vi "SearchGlyphs.vi"(4 "Glyphs tree":refnum<vi>, 6 "DNL_Glyphs []":refnum<vi>, 7 "Reset position? (F)":bool, 8 "error in (no error)":errorcluster, 10 "Keyword":string, 11 "Glyph in":refnum<class "Glyph.lvclass">) -> (0 "error out":errorcluster, 3 "Glyph out":refnum<class "Glyph.lvclass">)   [LabVIEW 2020, in "Glyph.lvclass"]
uses:
  Glyph.lvclass
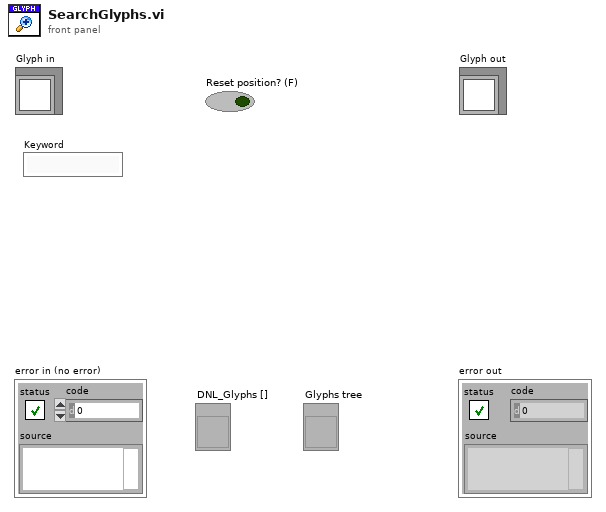
[diagram p1: front panel]
types:
  T1 = typedef "Graphic.ctl" = cluster{"Rectangle":cluster{"left":i16, "top":i16, "right":i16, "bottom":i16}, "Path":path, "Image":picture, "Filter":string, "FileName":string}
  T2 = typedef "Path&Icon.ctl" = cluster{"Rectangle":cluster{"left":i16, "top":i16, "right":i16, "bottom":i16}, "Path":path, "Image":picture, "Filter":string, "FileName":string}
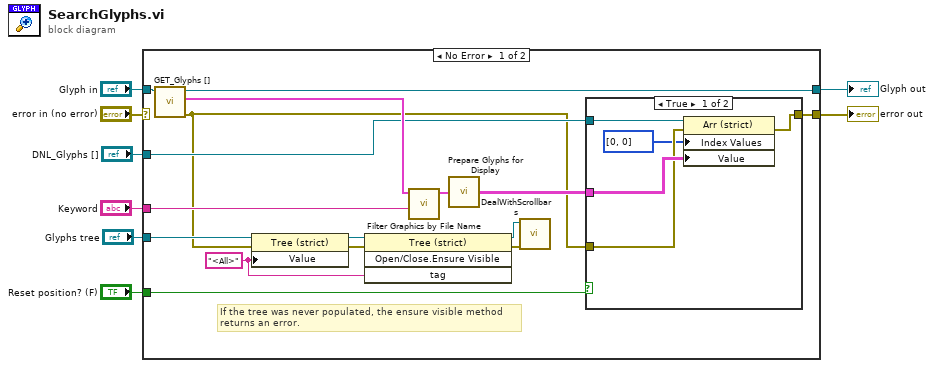
[diagram p0: block diagram]
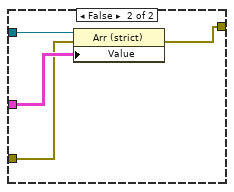
[diagram p2: hidden frame]
diagram:
  n1 = case shown="No Error" "error in (no error)" {
    selector: "error in (no error)" -> [_ w35]
    tunnel: [w22 w35] -> w7
    tunnel: [w23 w34] -> w5
    tunnel: "Glyph in" -> [w24 w34]
    tunnel: "Keyword" -> [w19 _]
    tunnel: "Reset position? (F)" -> [w17 _]
    tunnel: "Glyphs tree" -> [w16 _]
    tunnel: "DNL_Glyphs []" -> [w15 _]
    frame No Error {
      w10 = "<All>" ("Value")
      # "If the tree was never populated, the ensure visible method\nreturns an error."
      n2 = call-dynamic "GET_Glyphs [].vi"("Glyph.lvclass in"=w24) -> ("error out"=w9:errorcluster, "Glyphs []"=w20:T1[], "Glyph.lvclass out"=w23:refnum<class "Glyph.lvclass">)  [unwired: 1 in, 7 out]
      n3 = property class="Tree (strict)"(reference=w16, error in=w9, "Value"=w10) -> (reference out=w14:refnum<vi>, error out=w13:errorcluster)
      n4 = invoke class="Tree (strict)" method="Open/Close.Ensure Visible"(reference=w14, error in=w13, "tag"=w10) -> (reference out=w11:refnum<vi>, error out=w12:errorcluster)  [unwired: 1 in, 2 out]
      n5 = call "Filter Graphics by File Name.vi"("Keyword"=w19, "Icon Templates in"=w20) -> ("Icon Templates out"=w21:T2[])  [unwired: 9 out]
      n6 = call "Prepare Glyphs for Display.vi"("Icon Templates"=w21) -> ("Array"=w18:T2[][])
      n7 = call "DealWithScrollbars.vi"("error in (no error)"=w12, "Tree"=w11) -> ()  [unwired: 9 in, 1 out]
      n8 = case shown="True" w17 {
        tunnel: w15 -> [w29 w33]
        tunnel: [w28 w32] -> w22
        tunnel: w18 -> [w27 w31]
        tunnel: w9 -> [w26 w30]
        frame True {
          n9 = property class="Arr (strict)"(reference=w29, error in=w26, "Index Values"=u32[] [0, 0], "Value"=w27) -> (error out=w28:errorcluster)  [unwired: 1 out]
        }
        frame False {
          n10 = property class="Arr (strict)"(reference=w33, error in=w30, "Value"=w31) -> (error out=w32:errorcluster)  [unwired: 1 out]
        }
      }
    }
    frame Error {
    }
  }
  "error out" <- w7
  "Glyph out" <- w5
